vi "threshould calibration.vi"() -> ()   [LabVIEW 2019, in "Calibration Lib.lvlib"]
uses:
  Calibration Lib.lvlib
  <vilib>/Utility/miscctls.llb/LVRowAndColumnTypeDef.ctl
  <vilib>/addons/database/Connection.llb/DB Tools Open Connec (String).vi
  database.lvlib
  <vilib>/addons/database/NI_Database_API.lvlib
panel:
  in  "Delete":bool
  out "error out":errorcluster
  out "Error out":errorcluster
  out "data":string[][](array[string])
  out "Error out 3":errorcluster
  in  "Save":bool
  out "Calibration String":string
  in  "Close":bool
  in  "Calibrate":bool caption="Saving txt"
  out "Thresholds Table":string[][](table)
  in  "Disc Number":string(combo)
  out "Threshold 7":dbl
  out "Threshold 6":dbl
  out "Threshold 5":dbl
  out "Threshold 4":dbl
  out "Threshold 3":dbl
  out "Threshold 2":dbl
  out "Threshold 1":dbl caption="Threshoulds"
  in  ">18 mm":dbl
  in  "16-18 mm":dbl
  in  "14-16 mm":dbl
  in  "12.5-14 mm":dbl
  in  "10-12.5 mm":dbl
  in  "8-10 mm":dbl
  in  "6.3-8 mm":dbl
  in  "<6.3 mm":dbl caption="LAB RESULT"
  out "Threshoulds":dbl[](array[numeric])
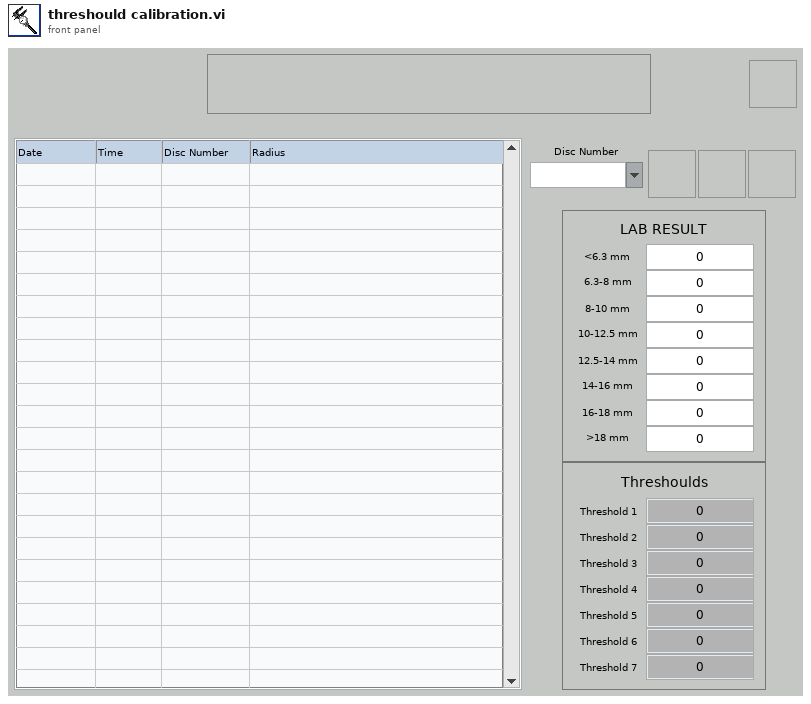
[diagram p1: front panel]
types:
  T1 = typedef "LVRowAndColumnTypeDef.ctl" = cluster{"Row":i32, "Column":i32}
  T2 = enum16{"None", "On Hover", "On Key Focus", "On Hover or Key Focus"}
  T3 = typedef "NI_Database_API.lvlib/Conn ObjectReference.ctl" = refnum<k1>
  T4 = cluster{string, string, string, string, string, string, string}
  T5 = cluster{i32, "date/time string":string, "date/time string":string, string}
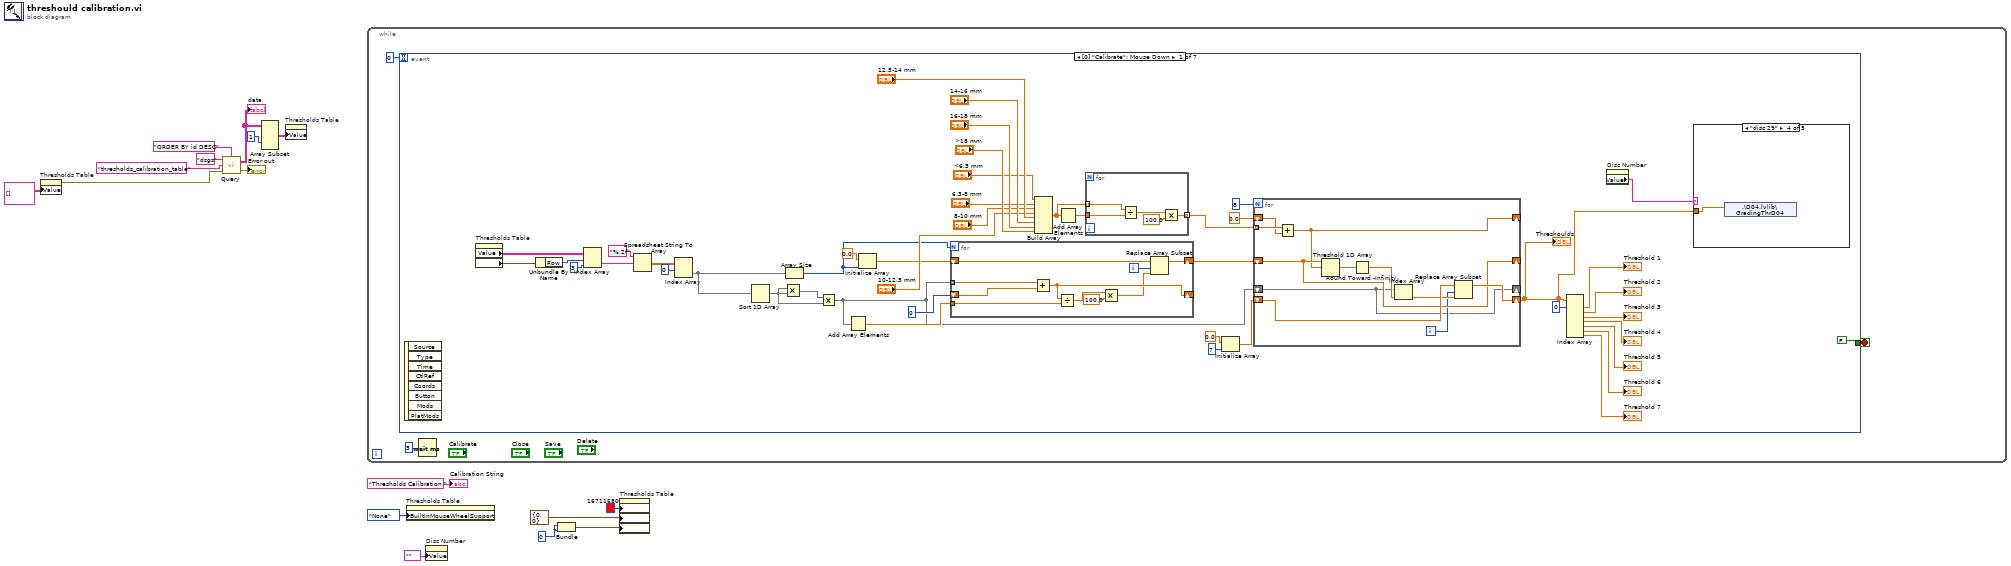
[diagram p0: block diagram]
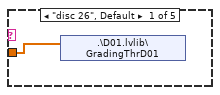
[diagram p2: hidden frame]
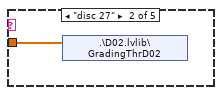
[diagram p3: hidden frame]
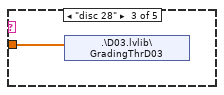
[diagram p4: hidden frame]
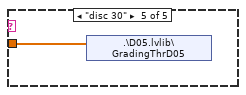
[diagram p5: hidden frame]
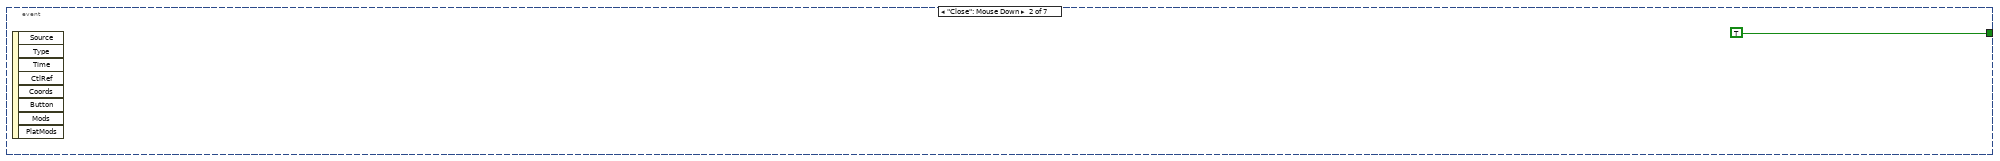
[diagram p6: hidden frame]
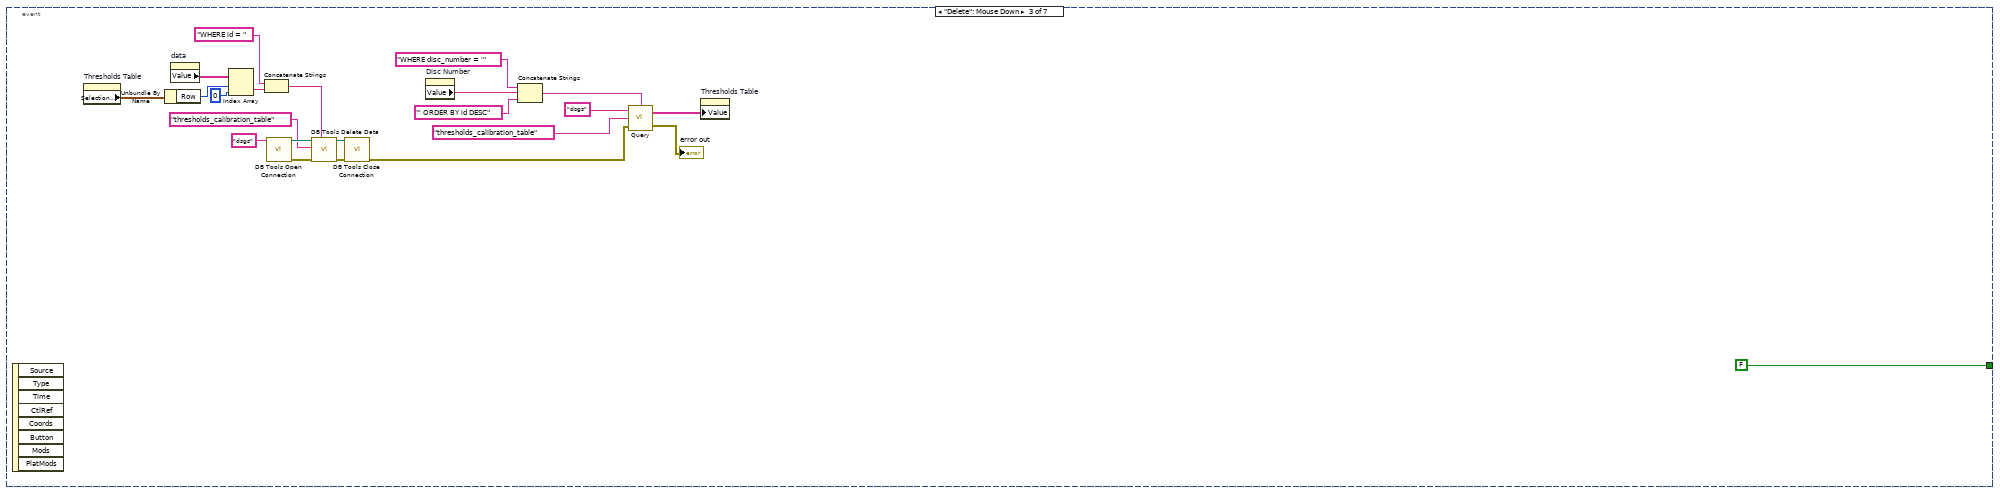
[diagram p7: hidden frame]
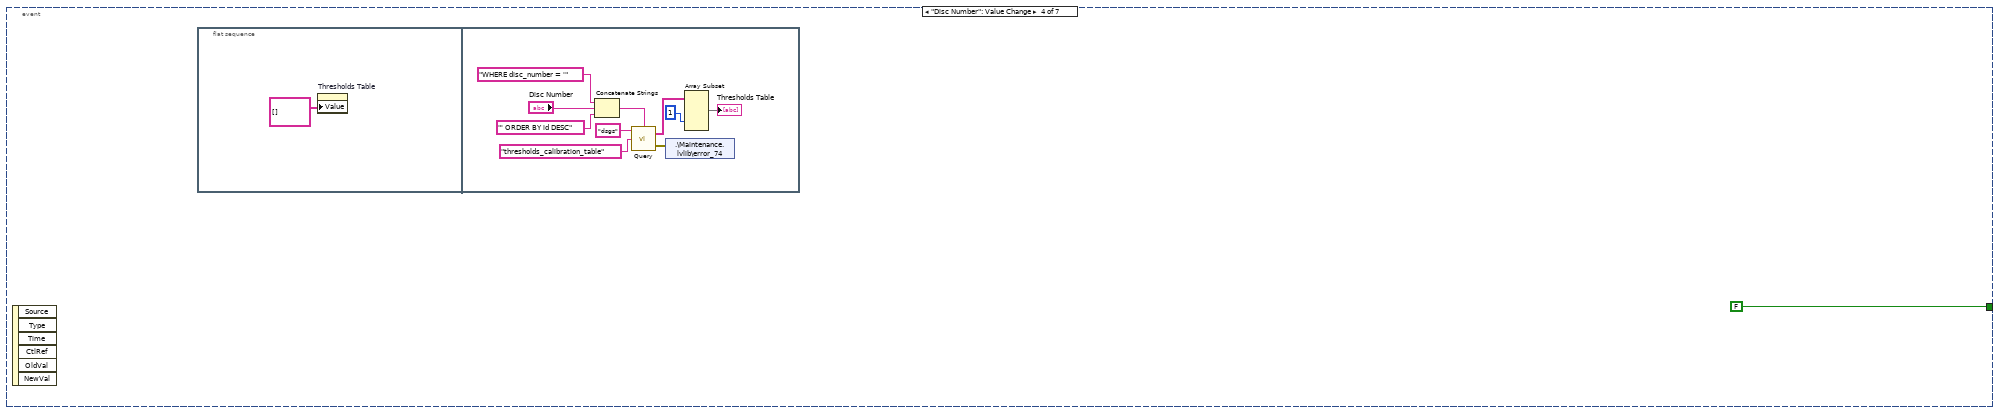
[diagram p8: hidden frame]
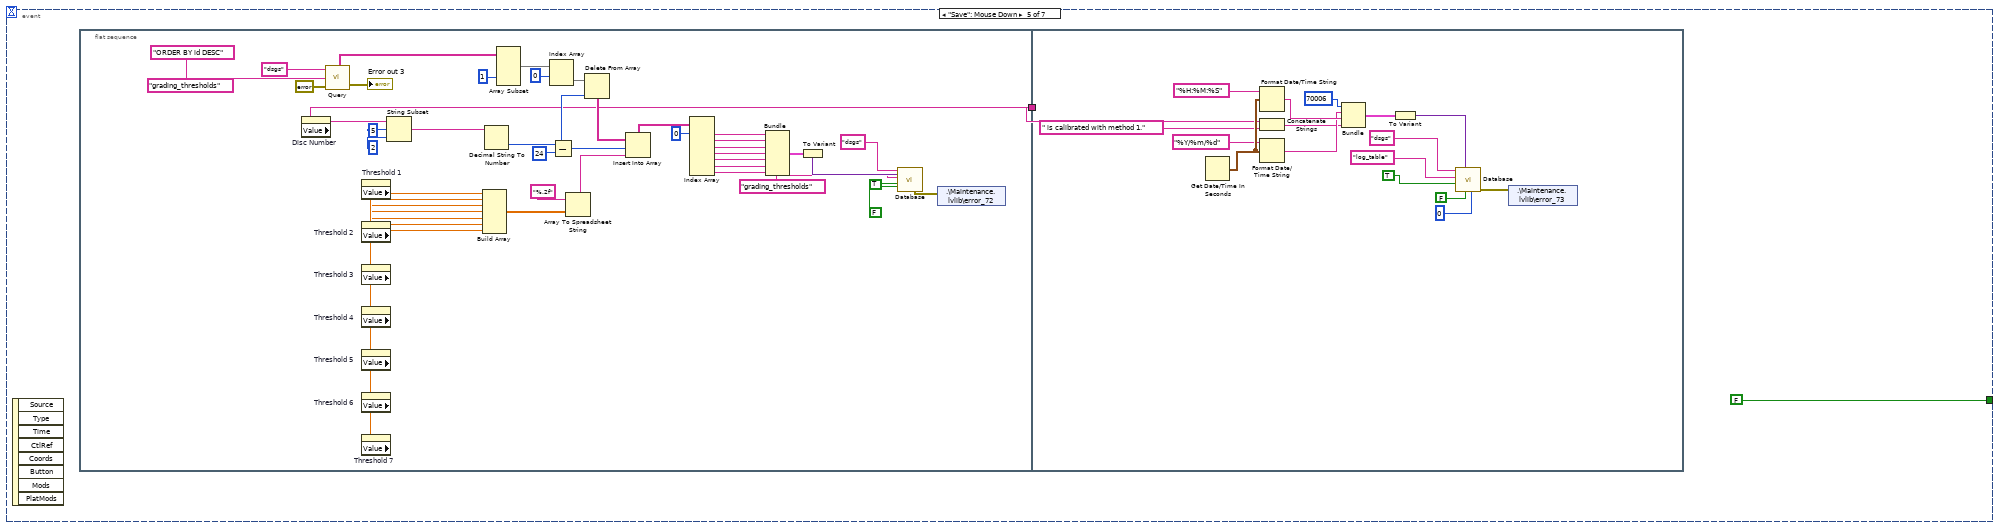
[diagram p9: hidden frame]
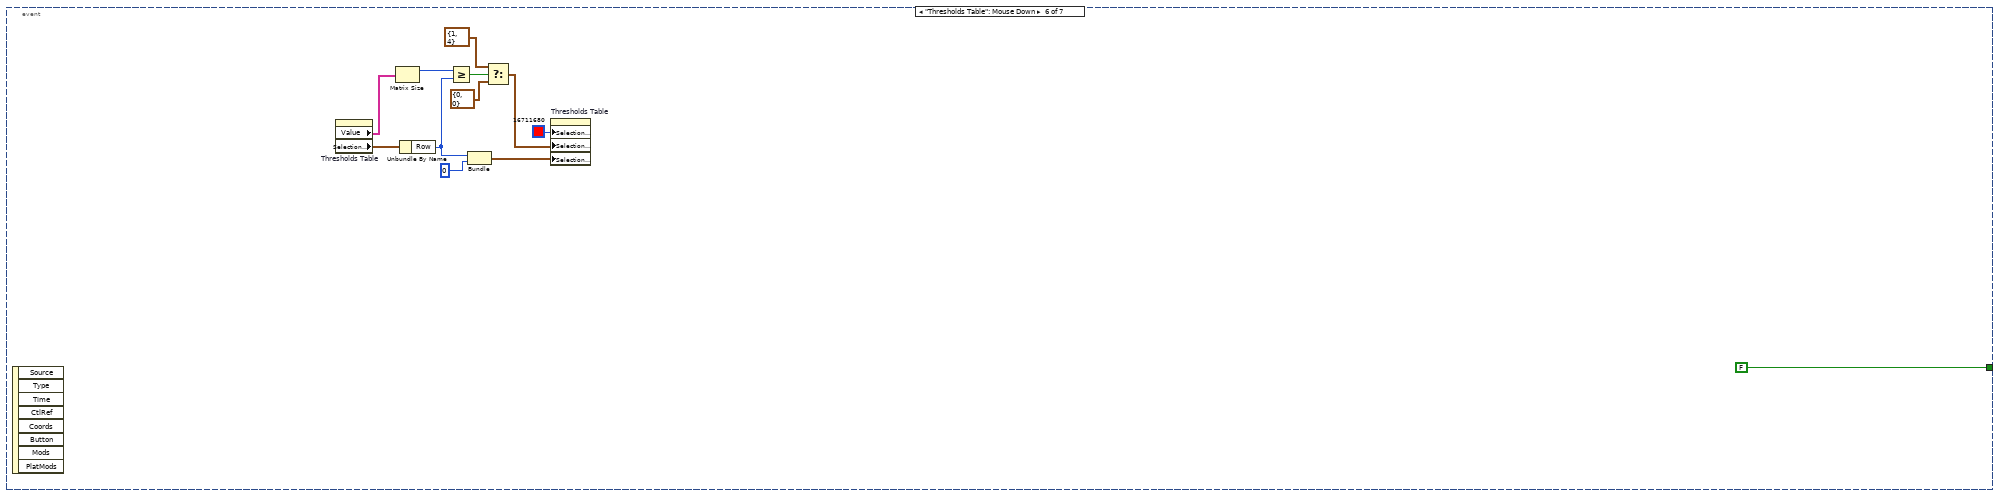
[diagram p10: hidden frame]
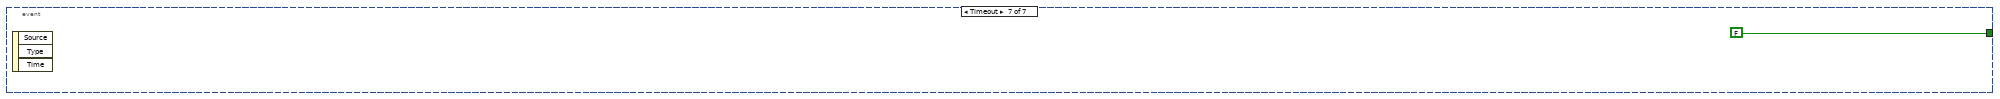
[diagram p11: hidden frame]
diagram:
  w4 = 0 ("Row")
  n1 = property on="Thresholds Table" class="Tbl (strict)"("Value"=string[][] [] ("Thresholds Table")) -> (error out=w1:errorcluster)  [unwired: 2 in, 1 out]
  n2 = call "Query.vi"("Condition"="ORDER BY id DESC", "Error in"=w1, "Table Name"="thresholds_calibration_table", "Connection Name"="dsgs") -> ("Error out"=→"Error out":errorcluster, "data"=w9:string[][])
  "data" <- w9
  n3 = Array Subset(array=w9, index (col)=1 ("index")) -> (w8:string[][])  [unwired: 3 in]
  n4 = property on="Thresholds Table" class="Tbl (strict)"("Value"=w8) -> ()  [unwired: 2 in, 2 out]
  n5 = while {
    stop <- w17 stop-if-true
    n6 = event shown="[0] \"Calibrate\": Mouse Down" {
      selector: _ -> [_ _ _ _ _ _ _]
      dyn-events: _ -> [_ _ _ _ _ _ _]
      timeout: 0 -> [_ _ _ _ _ _ _]
      tunnel: [FALSE TRUE FALSE FALSE FALSE FALSE FALSE] -> w17
      event "Calibrate": Mouse Down {
        n7 = event-data() -> ()  [unwired: 1 in, 8 out]
        n8 = property on="Thresholds Table" class="Tbl (strict)"() -> ("Value"=w61:string[][], "Selection Start"=w64:T1)  [unwired: 2 in, 2 out]
        n9 = Unbundle By Name(w64) -> ("Row"=w63:i32)
        n10 = Index Array(array=w61, index (row)=w63, index (col)=3 ("disabled index (col)")) -> (element=w60:string)
        n11 = Spreadsheet String To Array(format string="%.2f", spreadsheet string=w60) -> (array=w24:dbl[][])  [unwired: 2 in]
        n12 = Index Array(array=w24, index (row)=0 ("disabled index (col)")) -> (element=w23:dbl[])  [unwired: 1 in]
        n13 = Sort 1D Array(array=w23) -> (sorted array=w29:dbl[])
        n14 = Multiply(x=w29, y=w29) -> (x*y=w30:dbl[])
        n15 = Array Size(array=w23) -> (size(s)=w39:i32)
        n16 = Multiply(x=w30, y=w29) -> (x*y=w28:dbl[])
        n17 = Add Array Elements(numeric array=w28) -> (sum=w37:dbl)
        n18 = Initialize Array(0.0 ("element"), w39) -> (w40:dbl[])
        n19 = for {
          N: w39 -> [_]
          shift-right: [w91] -> w36
          shift-left: w40 -> [w93]
          tunnel: w28 -> [w95] mode=indexing
          shift-right: [w90] -> _
          shift-left: 0 ("disabled index (col)") -> [w94]
          tunnel: w37 -> [w89]
          i -> [w92]
          n20 = Add(x=w95, y=w94) -> (x+y=w90:dbl)
          n21 = Divide(x=w90, y=w89) -> (x/y=w88:dbl)
          n22 = Multiply(x=w88, y=100.0) -> (x*y=w86:dbl)
          n23 = Replace Array Subset(array=w93, new element=w86, index=w92) -> (w91:dbl[])
        }
        n24 = Build Array("<6.3 mm", "6.3-8 mm", "8-10 mm", "10-12.5 mm", "12.5-14 mm", "14-16 mm", "16-18 mm", ">18 mm") -> (w51:dbl[])
        n25 = Add Array Elements(numeric array=w51) -> (sum=w27:dbl)
        n26 = for {
          tunnel: w51 -> [w74] mode=indexing
          tunnel: w27 -> [w73]
          tunnel: [w70] -> w26 mode=indexing
          n27 = Divide(x=w74, y=w73) -> (x/y=w72:dbl)
          n28 = Multiply(x=w72, y=100.0) -> (x*y=w70:dbl)
        }
        n29 = Initialize Array(0.0 ("element"), 7 ("dimension size")) -> (w32:dbl[])
        n30 = for {
          N: 8 -> [_]
          shift-right: [w80] -> _
          shift-left: w36 -> [w80]
          tunnel: w26 -> [w79] mode=indexing
          shift-right: [w81] -> w20
          shift-left: w32 -> [w83]
          shift-right: [w77] -> _
          shift-left: 0.0 ("element") -> [w78]
          shift-right: [w75] -> _
          shift-left: w28 -> [w75]
          i -> [w76]
          n31 = Add(x=w79, y=w78) -> (x+y=w77:dbl)
          n32 = Threshold 1D Array(2:w77, 3:w80) -> (0:w85:dbl)  [unwired: 1 in]
          n33 = Round Toward -Infinity(1:w85) -> (0:w84:dbl)
          n34 = Index Array(array=w75, index=w84) -> (element=w82:dbl)
          n35 = Replace Array Subset(array=w83, new element=w82, index=w76) -> (w81:dbl[])
        }
        "Threshoulds" <- w20
        n36 = Index Array(array=w20, index #1=0 ("index")) -> (element #1=→"Threshold 1":dbl, element #2=→"Threshold 2":dbl, element #3=→"Threshold 3":dbl, element #4=→"Threshold 4":dbl, element #5=→"Threshold 5":dbl, element #6=→"Threshold 6":dbl, element #7=→"Threshold 7":dbl)  [unwired: 6 in]
        n37 = property on="Disc Number" class="CmbBox"() -> ("Value"=w21:string)  [unwired: 2 in, 2 out]
        n38 = case shown="\"disc 29\"" w21 {
          tunnel: w20 -> [w65 w66 w67 w68 w69]
          frame "disc 26", Default {
            n39 = shared-variable ".\\D01.lvlib\\GradingThrD01"(w65) -> ()  [unwired: 1 in, 1 out]
          }
          frame "disc 27" {
            n40 = shared-variable ".\\D02.lvlib\\GradingThrD02"(w66) -> ()  [unwired: 1 in, 1 out]
          }
          frame "disc 28" {
            n41 = shared-variable ".\\D03.lvlib\\GradingThrD03"(w67) -> ()  [unwired: 1 in, 1 out]
          }
          frame "disc 29" {
            n42 = shared-variable ".\\D04.lvlib\\GradingThrD04"(w68) -> ()  [unwired: 1 in, 1 out]
          }
          frame "disc 30" {
            n43 = shared-variable ".\\D05.lvlib\\GradingThrD05"(w69) -> ()  [unwired: 1 in, 1 out]
          }
        }
      }
      event "Close": Mouse Down {
        n44 = event-data() -> ()  [unwired: 1 in, 8 out]
      }
      event "Delete": Mouse Down {
        n45 = event-data() -> ()  [unwired: 1 in, 8 out]
        n46 = property on="Thresholds Table" class="Tbl (strict)"() -> ("Selection Start"=w113:T1)  [unwired: 2 in, 2 out]
        n47 = Unbundle By Name(w113) -> ("Row"=w111:i32)
        n48 = property on="data" class="Arr (strict)"() -> ("Value"=w112:string[][])  [unwired: 2 in, 2 out]
        n49 = Index Array(array=w112, index (row)=w111, index (col)=0 ("disabled index (col)")) -> (element=w116:string)
        n50 = Concatenate Strings("WHERE id = " ("string"), w116) -> (w117:string)
        n51 = call-poly <vilib>:"DB Tools Open Connection.vi"("connection information"="dsgs") -> ("error out"=w115:errorcluster, "connection reference"=w114:T3)  [unwired: 7 in]
        n52 = call <vilib>:"DB Tools Delete Data.vi"("condition"=w117, "error in (no error)"=w115, "table"="thresholds_calibration_table", "connection reference"=w114) -> ("error out"=w118:errorcluster, "connection reference out"=w119:T3)  [unwired: 6 in]
        n53 = call <vilib>:"DB Tools Close Connection.vi"("error in (no error)"=w118, "connection reference"=w119) -> ("error out"=w101:errorcluster)  [unwired: 5 in]
        n54 = property on="Disc Number" class="CmbBox"() -> ("Value"=w99:string)  [unwired: 2 in, 2 out]
        n55 = Concatenate Strings("WHERE disc_number = '", w99, "' ORDER BY id DESC" ("string")) -> (w106:string)
        n56 = call "Query.vi"("Condition"=w106, "Error in"=w101, "Table Name"="thresholds_calibration_table", "Connection Name"="dsgs") -> ("Error out"=→"error out":errorcluster, "data"=w98:string[][])
        n57 = property on="Thresholds Table" class="Tbl (strict)"("Value"=w98) -> ()  [unwired: 2 in, 2 out]
      }
      event "Disc Number": Value Change {
        n58 = event-data() -> ()  [unwired: 1 in, 6 out]
        n59 = flat-sequence {
          frame #0 {
            n60 = property on="Thresholds Table" class="Tbl (strict)"("Value"=string[][] [] ("Thresholds Table")) -> ()  [unwired: 2 in, 2 out]
          }
          frame #1 {
            n61 = Concatenate Strings("WHERE disc_number = '", "Disc Number", "' ORDER BY id DESC" ("string")) -> (w129:string)
            n62 = call "Query.vi"("Condition"=w129, "Table Name"="thresholds_calibration_table", "Connection Name"="dsgs") -> ("Error out"=w122:errorcluster, "data"=w130:string[][])  [unwired: 1 in]
            n63 = shared-variable ".\\Maintenance.lvlib\\error_74"(w122) -> ()  [unwired: 1 in, 1 out]
            n64 = Array Subset(array=w130, index (col)=1 ("index")) -> (→"Thresholds Table":string[][])  [unwired: 3 in]
          }
        }
      }
      event "Save": Mouse Down {
        n65 = event-data() -> ()  [unwired: 1 in, 8 out]
        n66 = flat-sequence {
          tunnel: [w135] -> w132
          tunnel: w132 -> [w179]
          frame #0 {
            n67 = property on="Disc Number" class="CmbBox"() -> ("Value"=w135:string)  [unwired: 2 in, 2 out]
            n68 = call "Query.vi"("Condition"="ORDER BY id DESC", "Error in"=errorcluster {"status"=FALSE, "code"=0, "source"=""}, "Table Name"="grading_thresholds", "Connection Name"="dsgs") -> ("Error out"=→"Error out 3":errorcluster, "data"=w167:string[][])
            n69 = property on="Threshold 1" class="DigNum (strict)"() -> ("Value"=w154:dbl)  [unwired: 2 in, 2 out]
            n70 = property on="Threshold 2" class="DigNum (strict)"() -> ("Value"=w153:dbl)  [unwired: 2 in, 2 out]
            n71 = property on="Threshold 3" class="DigNum (strict)"() -> ("Value"=w152:dbl)  [unwired: 2 in, 2 out]
            n72 = property on="Threshold 4" class="DigNum (strict)"() -> ("Value"=w151:dbl)  [unwired: 2 in, 2 out]
            n73 = property on="Threshold 5" class="DigNum (strict)"() -> ("Value"=w150:dbl)  [unwired: 2 in, 2 out]
            n74 = property on="Threshold 6" class="DigNum (strict)"() -> ("Value"=w149:dbl)  [unwired: 2 in, 2 out]
            n75 = property on="Threshold 7" class="DigNum (strict)"() -> ("Value"=w148:dbl)  [unwired: 2 in, 2 out]
            n76 = String Subset(string=w135, offset (0)=5, length (rest)=2 ("length (rest)")) -> (substring=w172:string)
            n77 = Build Array(w154, w153, w152, w151, w150, w149, w148) -> (w147:dbl[])
            n78 = Decimal String To Number(string=w172) -> (number=w171:i32)  [unwired: 2 in, 1 out]
            n79 = Array Subset(array=w167, index (col)=1 ("index")) -> (w166:string[][])  [unwired: 3 in]
            n80 = Index Array(array=w166, index (row)=0) -> (element=w164:string[])  [unwired: 1 in]
            n81 = Subtract(x=w171, y=24) -> (x-y=w162:i32)
            n82 = Array To Spreadsheet String(array=w147, 3:"%.2f" ("format string")) -> (spreadsheet string=w160:string)  [unwired: 1 in]
            n83 = Delete From Array(array=w164, index=w162) -> (array with subset deleted=w163:string[])  [unwired: 1 in, 1 out]
            n84 = Insert Into Array(array=w163, index=w162, new element=w160) -> (w146:string[])
            n85 = Index Array(array=w146, index #1=0 ("index")) -> (element #1=w138:string, element #2=w139:string, element #3=w140:string, element #4=w141:string, element #5=w142:string, element #6=w143:string, element #7=w144:string)  [unwired: 6 in]
            n86 = Bundle(w138, w139, w140, w141, w142, w143, w144) -> (w137:T4)  [unwired: 1 in]
            n87 = To Variant(anything=w137) -> (Variant=w159:variant)
            n88 = call "Database.vi"("Delete row?"=FALSE, "Data"=w159, "Auto Increment ID?"=TRUE, "Table"="grading_thresholds", "Connection"="dsgs") -> ("Error out"=w134:errorcluster)  [unwired: 6 in]
            n89 = shared-variable ".\\Maintenance.lvlib\\error_72"(w134) -> ()  [unwired: 1 in, 1 out]
          }
          frame #1 {
            n90 = Get Date/Time In Seconds() -> (seconds since 1Jan1904=w190:timestamp)
            n91 = Format Date/Time String(time format string (%c)="%H:%M:%S", seconds (now)=w190) -> (date/time string=w192:string)  [unwired: 1 in]
            n92 = Concatenate Strings(w179, " is calibrated with method 1." ("string")) -> (w180:string)
            n93 = Format Date/Time String(time format string (%c)="%Y/%m/%d", seconds (now)=w190) -> (date/time string=w191:string)  [unwired: 1 in]
            n94 = Bundle(70006, "date/time string"=w191, "date/time string"=w192, w180) -> (w193:T5)  [unwired: 1 in]
            n95 = To Variant(anything=w193) -> (Variant=w194:variant)
            n96 = call "Database.vi"("Maximum Row"=u64 0 ("Storage Time (Day)"), "Delete row?"=FALSE, "Data"=w194, "Auto Increment ID?"=TRUE, "Table"="log_table" ("table"), "Connection"="dsgs" ("table")) -> ("Error out"=w178:errorcluster)  [unwired: 5 in]
            n97 = shared-variable ".\\Maintenance.lvlib\\error_73"(w178) -> ()  [unwired: 1 in, 1 out]
          }
        }
      }
      event "Thresholds Table": Mouse Down {
        n98 = event-data() -> ()  [unwired: 1 in, 8 out]
        n99 = property on="Thresholds Table" class="Tbl (strict)"() -> ("Value"=w202:string[][], "Selection Start"=w206:T1)  [unwired: 2 in, 2 out]
        n100 = Matrix Size(0:w202) -> (1:w200:i32)  [unwired: 1 out]
        n101 = Unbundle By Name(w206) -> ("Row"=w201:i32)
        n102 = Greater Or Equal?(x=w200, y=w201) -> (x >= y?=w199:bool)
        n103 = Bundle("Row"=w201, "Row"=0) -> (w204:cluster{"Row":i32, "Row":i32})  [unwired: 1 in]
        n104 = Select(t=T1 {"Row"=1, "Column"=4} ("Selection Size"), s=w199, f=T1 {"Row"=0, "Column"=0}) -> (s? t:f=w196:T1)
        n105 = property on="Thresholds Table" class="Tbl (strict)"("Selection Color"=u32 16711680, "Selection Size"=w196, "Selection Start"=w204) -> ()  [unwired: 2 in, 2 out]
      }
      event Timeout {
        n106 = event-data() -> ()  [unwired: 1 in, 3 out]
      }
    }
    n107 = Wait (ms)(milliseconds to wait=u32 5) -> ()  [unwired: 1 out]
  }
  n108 = property on="Thresholds Table" class="Tbl (strict)"("BuiltInMouseWheelSupport"=T2."None" ("Built-In Mouse Wheel Support")) -> ()  [unwired: 2 in, 2 out]
  n109 = property on="Disc Number" class="CmbBox"("Value"="" ("Disc Number")) -> ()  [unwired: 2 in, 2 out]
  n110 = Bundle("Row"=w4, "Row"=w4) -> (w7:cluster{"Row":i32, "Row":i32})  [unwired: 1 in]
  n111 = property on="Thresholds Table" class="Tbl (strict)"("Selection Color"=u32 16711680, "Selection Size"=T1 {"Row"=0, "Column"=0} ("f"), "Selection Start"=w7) -> ()  [unwired: 2 in, 2 out]
  "Calibration String" <- "Thresholds Calibration " ("Calibration String")
